vi "Read T.vi"(8 "error in (no error)":errorcluster, 11 "Domain_Evolut.lvclass in":refnum<class "NI_Domain_Evolut.lvclass">) -> (0 "error out":errorcluster, 2 "t":T1, 3 "Domain_Evolut.lvclass out":refnum<class "NI_Domain_Evolut.lvclass">)   [LabVIEW 2017, in "NI_PDE.lvlib" / "NI_Domain_Evolut.lvclass"]
uses:
  <vilib>/gmath/pde.llb/DomainClass/Domain_Evolut/NI_Domain_Evolut.lvclass
  <vilib>/gmath/pde.llb/DomainClass/Domain_Evolut/NI_Domain_Evolut.lvclass/NI_Domain_Evolut.ctl
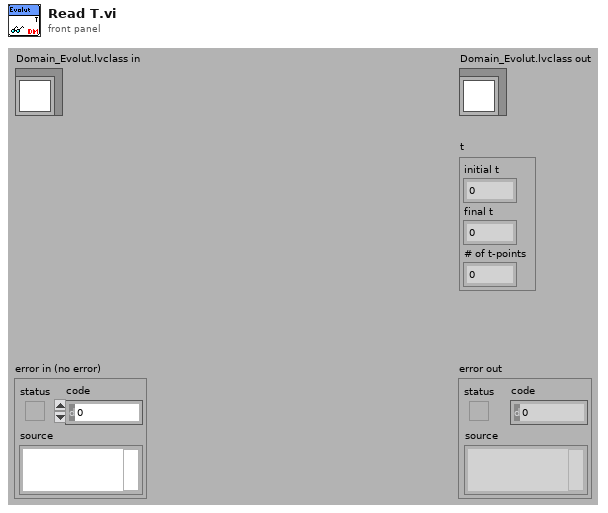
[diagram p1: front panel]
types:
  T1 = cluster{"initial t":dbl, "final t":dbl, "# of t-points":i32}
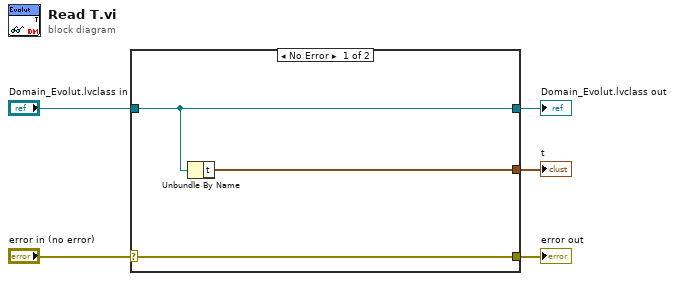
[diagram p0: block diagram]
diagram:
  n1 = case shown="No Error" "error in (no error)" {
    selector: "error in (no error)" -> [w8 w9]
    tunnel: [w8 w9] -> w4
    tunnel: [w7 w10] -> w2
    tunnel: "Domain_Evolut.lvclass in" -> [w7 w10]
    tunnel: [w6 _] -> w1
    frame No Error {
      n2 = Unbundle By Name(w7) -> ("t"=w6:T1)
    }
    frame Error {
    }
  }
  "error out" <- w4
  "Domain_Evolut.lvclass out" <- w2
  "t" <- w1
